vi "修改数据发送起始时间.vi"() -> ()   [LabVIEW 2016]
uses:
  <vilib>/Utility/config.llb/NI_LVConfig.lvlib
panel:
  in  "确定":bool caption="返回"
  in  "返回":bool
  in  "时间标识":timestamp
  # "修改数据发送起始时间"
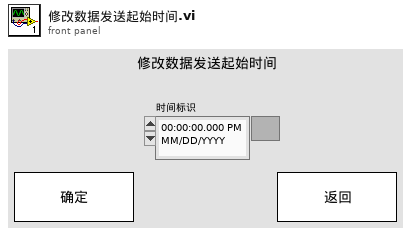
[diagram p1: front panel]
types:
  T1 = cluster{"time1":string, "time2":string, "time3":string, "time4":string, "time5":string, "time6":string, "time7":string, "time8":string, "time9":string, "time10":string, "time11":string, "time12":string, "time13":string, "time14":string, "time15":string, "time16":string, "time17":string, "time18":string, "time19":string, "time20":string, "time21":string, "time22":string, "time23":string, "time24":string, "time25":string, "time26":string, "time27":string, "time28":string, "time29":string, "time30":string, "time31":string}
  T2 = cluster{"[0]":string, "[1]":string, "[2]":string, "[3]":string, "[4]":string, "[5]":string, "[6]":string, "[7]":string, "[8]":string, "[9]":string, "[10]":string, "[11]":string, "[12]":string, "[13]":string, "[14]":string, "[15]":string, "[16]":string, "[17]":string, "[18]":string, "[19]":string, "[20]":string, "[21]":string, "[22]":string, "[23]":string, "[24]":string, "[25]":string, "[26]":string, "[27]":string, "[28]":string, "[29]":string, "[30]":string}
  T3 = typedef "NI_LVConfig.lvlib/Config Data RefNum.ctl" = refnum<k1>
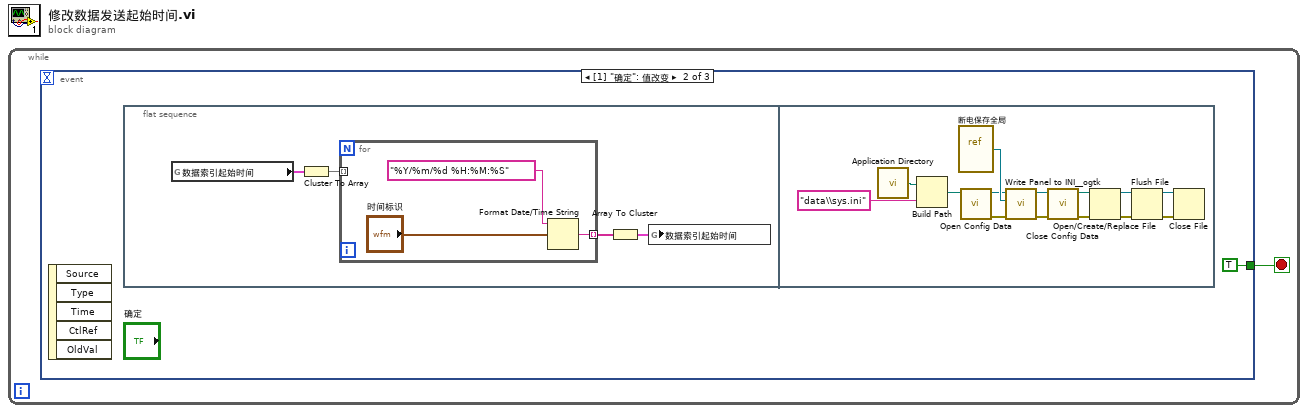
[diagram p0: block diagram]
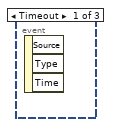
[diagram p2: hidden frame]
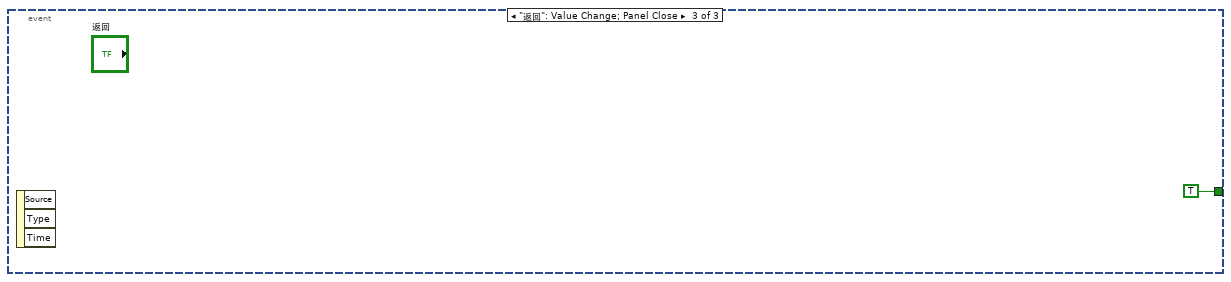
[diagram p3: hidden frame]
diagram:
  n1 = while {
    stop <- w1 stop-if-true
    n2 = event shown="[1] \"确定\": 值改变" {
      selector: _ -> [_ _ _]
      dyn-events: _ -> [_ _ _]
      timeout: _ -> [_ _ _]
      tunnel: [_ TRUE TRUE] -> w1
      event Timeout {
        n3 = event-data() -> ()  [unwired: 1 in, 3 out]
      }
      event "确定": Value Change {
        n4 = event-data() -> ()  [unwired: 1 in, 5 out]
        n5 = flat-sequence {
          frame #0 {
            n6 = global read "内部全局.vi" "数据索引起始时间"() -> (w5:T1)
            n7 = Cluster To Array(cluster=w5) -> (array=w4:string[])
            n8 = for {
              tunnel: w4 -> [_] mode=indexing
              tunnel: [w7] -> w3 mode=indexing
              n9 = Format Date/Time String(time format string (%c)="%Y/%m/%d %H:%M:%S" ("时间格式字符串(%c)"), seconds (now)="时间标识") -> (date/time string=w7:string)  [unwired: 1 in]
            }
            n10 = Array To Cluster(array=w3) -> (cluster=w6:T2)
            n11 = global write "内部全局.vi" "数据索引起始时间"(w6) -> ()
          }
          frame #1 {
            n12 = call <vilib>:"Application Directory.vi"() -> ("Application Directory"=w10:path)
            n13 = Build Path(base path=w10, name or relative path="data\\sys.ini" ("名称或相对路径")) -> (appended path=w12:path)
            n14 = vi-ref "断电保存全局.vi"() -> (w14:refnum<vi>)
            n15 = call <vilib>:"Open Config Data.vi"("configuration file path"=w12) -> ("error out"=w16:errorcluster, "refnum"=w13:T3)  [unwired: 8 in, 1 out]
            n16 = call <userlib>:"Write Panel to INI__ogtk.vi"("error in (no error)"=w16, "VI ref"=w14, "refnum"=w13) -> ("error out"=w17:errorcluster, "refnum out"=w15:T3)  [unwired: 7 in]
            n17 = call <vilib>:"Close Config Data.vi"("error in (no error)"=w17, "refnum"=w15) -> ("error out"=w22:errorcluster, "file path"=w23:path)  [unwired: 8 in]
            n18 = Open/Create/Replace File(file path (use dialog)=w23, error in=w22) -> (refnum out=w19:refnum<file>, error out=w18:errorcluster)  [unwired: 4 in, 1 out]
            n19 = Flush File(refnum=w19, error in=w18) -> (refnum out=w20:refnum<file>, error out=w21:errorcluster)
            n20 = Close File(refnum=w20, error in=w21) -> ()  [unwired: 2 out]
          }
        }
      }
      event "返回": Value Change; Panel Close {
        n21 = event-data() -> ()  [unwired: 1 in, 3 out]
      }
    }
  }
